vi "Read Laser Control.vi"(8 "error in (no error)":errorcluster, 11 "Change PAS Laser Parameters in":refnum<class "Change PAS Laser Parameters.lvclass">) -> (0 "error out":errorcluster, 2 "Laser Control":T1 {"Vrange" min=0 max=20}, 3 "Change PAS Laser Parameters out":refnum<class "Change PAS Laser Parameters.lvclass">)   [LabVIEW 2014, in "Change PAS Laser Parameters.lvclass"]
uses:
  Change PAS Laser Parameters.lvclass
  Change PAS Laser Parameters.lvclass/Change PAS Laser Parameters.ctl
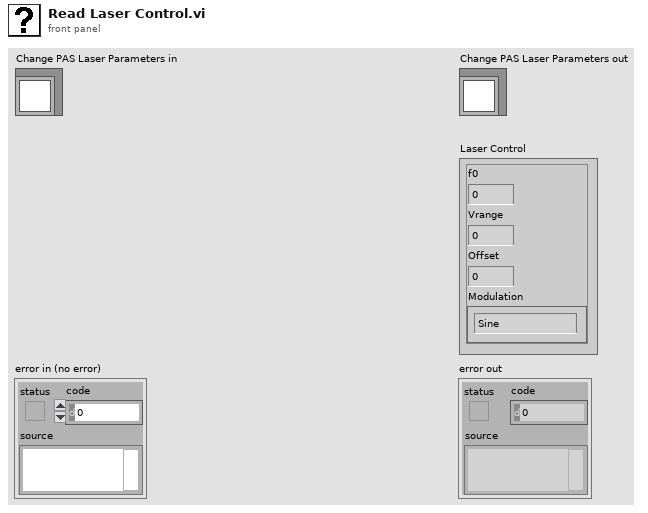
[diagram p1: front panel]
types:
  T1 = cluster{"f0":u16, "Vrange":sgl, "Offset":sgl, "Modulation":enum8{"Sine", "Square"}}
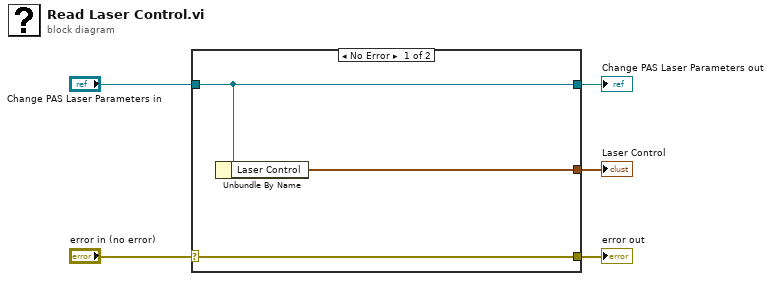
[diagram p0: block diagram]
diagram:
  n1 = case shown="No Error" "error in (no error)" {
    selector: "error in (no error)" -> [w8 w9]
    tunnel: [w8 w9] -> w4
    tunnel: [w7 w10] -> w2
    tunnel: "Change PAS Laser Parameters in" -> [w7 w10]
    tunnel: [w6 _] -> w1
    frame No Error {
      n2 = Unbundle By Name(w7) -> ("Laser Control"=w6:T1)
    }
    frame Error {
    }
  }
  "error out" <- w4
  "Change PAS Laser Parameters out" <- w2
  "Laser Control" <- w1
